vi "InjectPoints.vi"(10 "Spacing":dbl, 11 "Path":cluster{"x":dbl, "y":dbl}[](array[cluster])) -> (3 "Path out":cluster{dbl, dbl}[](array[cluster]))   [LabVIEW 2018]
doc: "Inserts points into a path with a certain spacing."
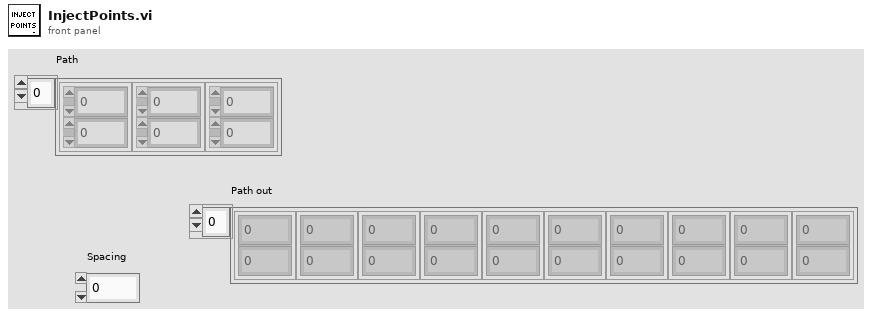
[diagram p1: front panel]
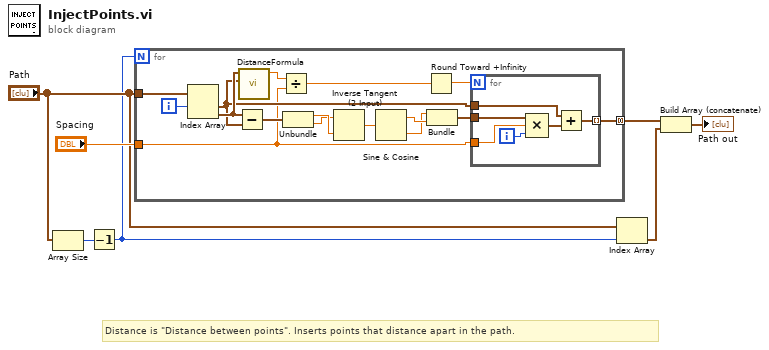
[diagram p0: block diagram]
diagram:
  # "Distance is \"Distance between points\". Inserts points that distance apart in the path."
  n1 = Array Size(array="Path") -> (size(s)=w7:i32)
  n2 = Decrement(x=w7) -> (x-1=w2:i32)
  n3 = for {
    N: w2 -> [_]
    tunnel: "Path" -> [w23]
    tunnel: "Spacing" -> [w12]
    tunnel: [w8] -> w5 mode=concatenating
    i -> [w22]
    n4 = Index Array(array=w23, index #1=w22) -> (element #1=w14:cluster{"x":dbl, "y":dbl}, element #2=w15:cluster{"x":dbl, "y":dbl})  [unwired: 1 in]
    n5 = Subtract(x=w15, y=w14) -> (x-y=w21:cluster{"x":dbl, "y":dbl})
    n6 = call "DistanceFormula.vi"("Point 2"=w14, "Point 1"=w15) -> ("Distance"=w13:dbl)  [unwired: 9 in]
    n7 = Divide(x=w13, y=w12) -> (x/y=w10:dbl)
    n8 = Unbundle(w21) -> ("x"=w20:dbl, "y"=w19:dbl)
    n9 = Inverse Tangent (2 Input)(1:w20, 2:w19) -> (0:w18:dbl)
    n10 = Sine & Cosine(0:w18) -> (1:w17:dbl, 2:w16:dbl)
    n11 = Round Toward +Infinity(x=w10) -> (ceil(x): smallest int >= x=w9:dbl)
    n12 = Bundle(w16, w17) -> (w11:cluster{dbl, dbl})  [unwired: 1 in]
    n13 = for {
      N: w9 -> [_]
      tunnel: w14 -> [w29]
      tunnel: w11 -> [w25]
      tunnel: [w28] -> w8 mode=indexing
      tunnel: w12 -> [w26]
      i -> [w27]
      n14 = Compound Arithmetic op=MULTIPLY(w25, w26, w27) -> (w24:cluster{dbl, dbl})
      n15 = Add(x=w29, y=w24) -> (x+y=w28:cluster{dbl, dbl})
    }
  }
  n16 = Index Array(array="Path", index=w2) -> (element=w1:cluster{"x":dbl, "y":dbl})
  n17 = Build Array (concatenate)(w5, w1) -> (→"Path out":cluster{"x":dbl, "y":dbl}[])
